vi "ma_sml_Window Frequency Response (double array).vi"(1 "N (window length)":i32=512, 2 "window":u16(ring) items=["Rectangle"=0, "Hanning"=1, "Hamming"=2, "Blackman-Harris"=3, "Exact Blackman"=4, "Blackman"=5, "Flat Top"=6, "4 Term B-Harris "=7, "7 Term B-Harris"=8, "Low Sidelobe"=9, "Blackman Nuttall"=11, "Triangle"=30, "Bartlett-Hanning"=31, "Bohman"=32, "Parzen"=33, "Welch"=34, "Kaiser"=60, "Dolph-Chebyshev"=61, "Gaussian"=62], 3 "f(normalized)":dbl[](array[numeric]) format="%.5f") -> (0 "H(f)":cdb[](array[numeric]) format="%.2f")   [LabVIEW 2020, in "NI_MAPro.lvlib"]
uses:
  NI_MAPro.lvlib
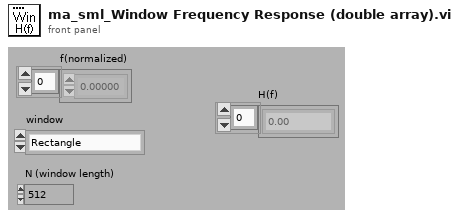
[diagram p1: front panel]
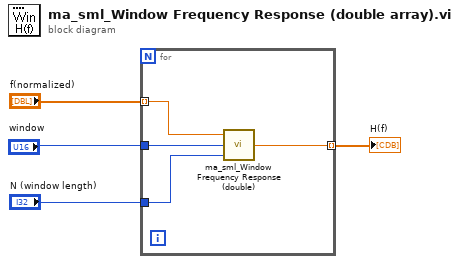
[diagram p0: block diagram]
diagram:
  n1 = for {
    tunnel: "f(normalized)" -> [w8] mode=indexing
    tunnel: "window" -> [w7]
    tunnel: "N (window length)" -> [w6]
    tunnel: [w5] -> w1 mode=indexing
    n2 = call "ma_sml_Window Frequency Response (double).vi"("N (window length)"=w6, "window"=w7, "f(normalized)"=w8) -> ("H(f)"=w5:cdb)
  }
  "H(f)" <- w1
